vi "analyze-single-vi.vi"(0 "GObj引用句柄":refnum<vi>, 1 "type":string="subvi", 2 "context":string[][](array[string]), 3 "json_input":string caption="<JSON>Object") -> (7 "<JSON> 3":string caption="<JSON>")   [LabVIEW 2020]
panel:
  out "VI路径":path
  out "所有对象[] 2":string[][](table)
  out "数组 2":string[](array[string])
  in  "字符串":string="data\\"
  out "添加的路径":path
  out "x > 0?":bool
  out "布尔":bool
  in  "路径":path=path "C:/Users/Fred/Desktop/LabAI"
  in  "排除路径":string[](array[string])=["E:\\LabVIEW\\32-bit\\LabVIEW 2020"]
  in  "Path to Entrance VI":path=path "C:/Users/Fred/Desktop/LabAI/main.vi"
  # "C:\\Users\\Fred\\Desktop\\LabAI\\get_status_code.vi"
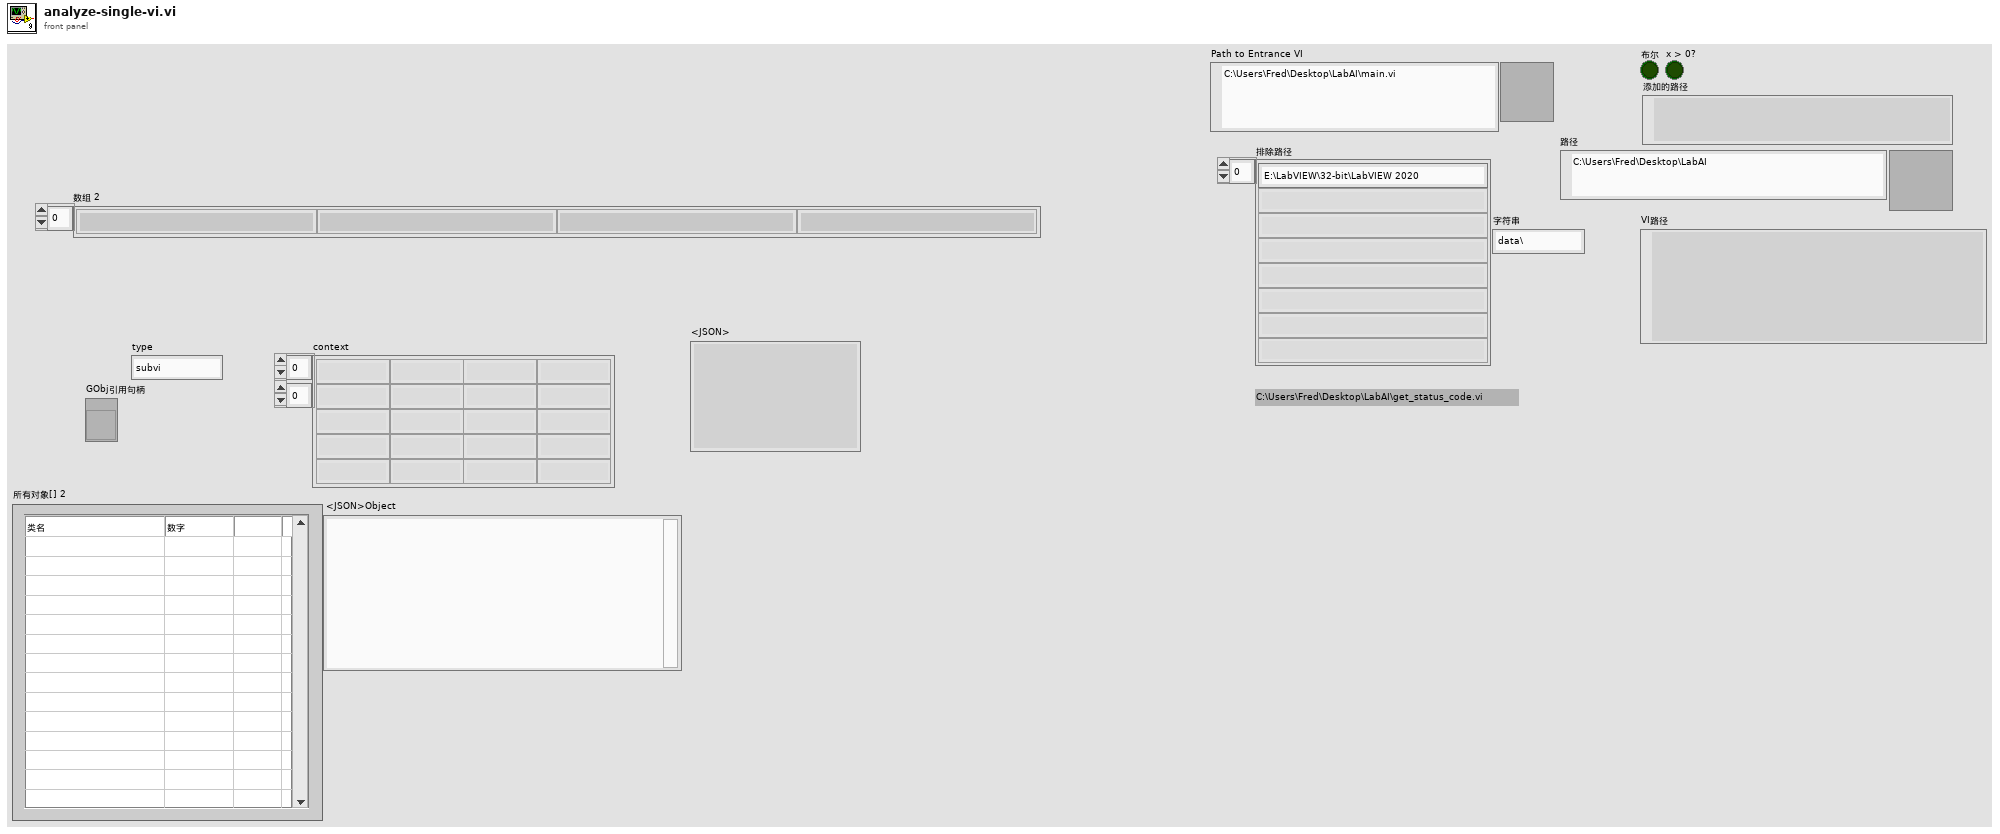
[diagram p1: front panel]
types:
  T1 = enum16{"open", "replace", "create", "open or create", "replace or create", "replace or create with confirmation"}
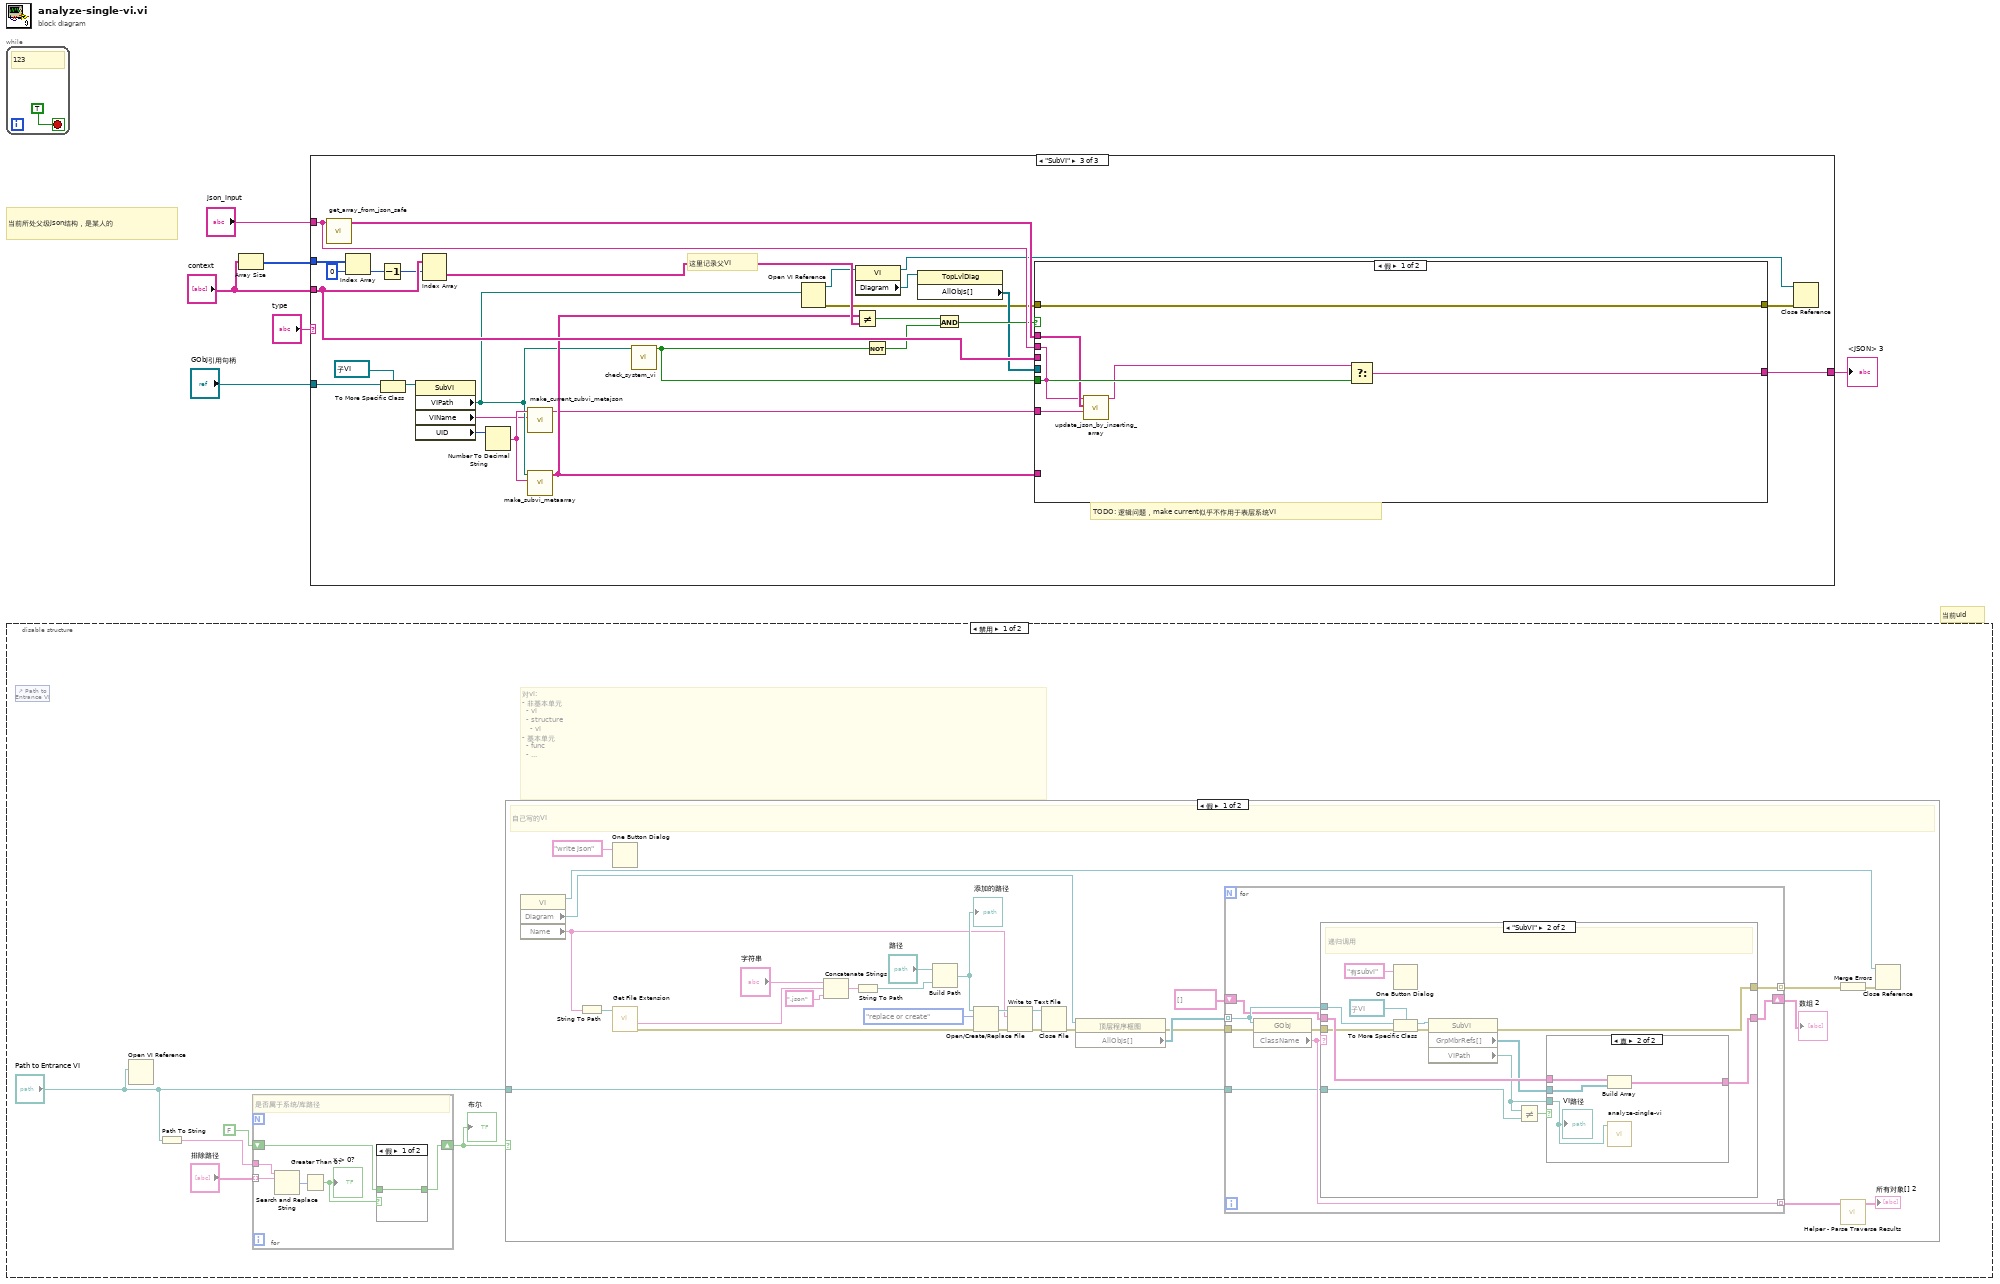
[diagram p0: block diagram]
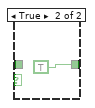
[diagram p2: hidden frame]
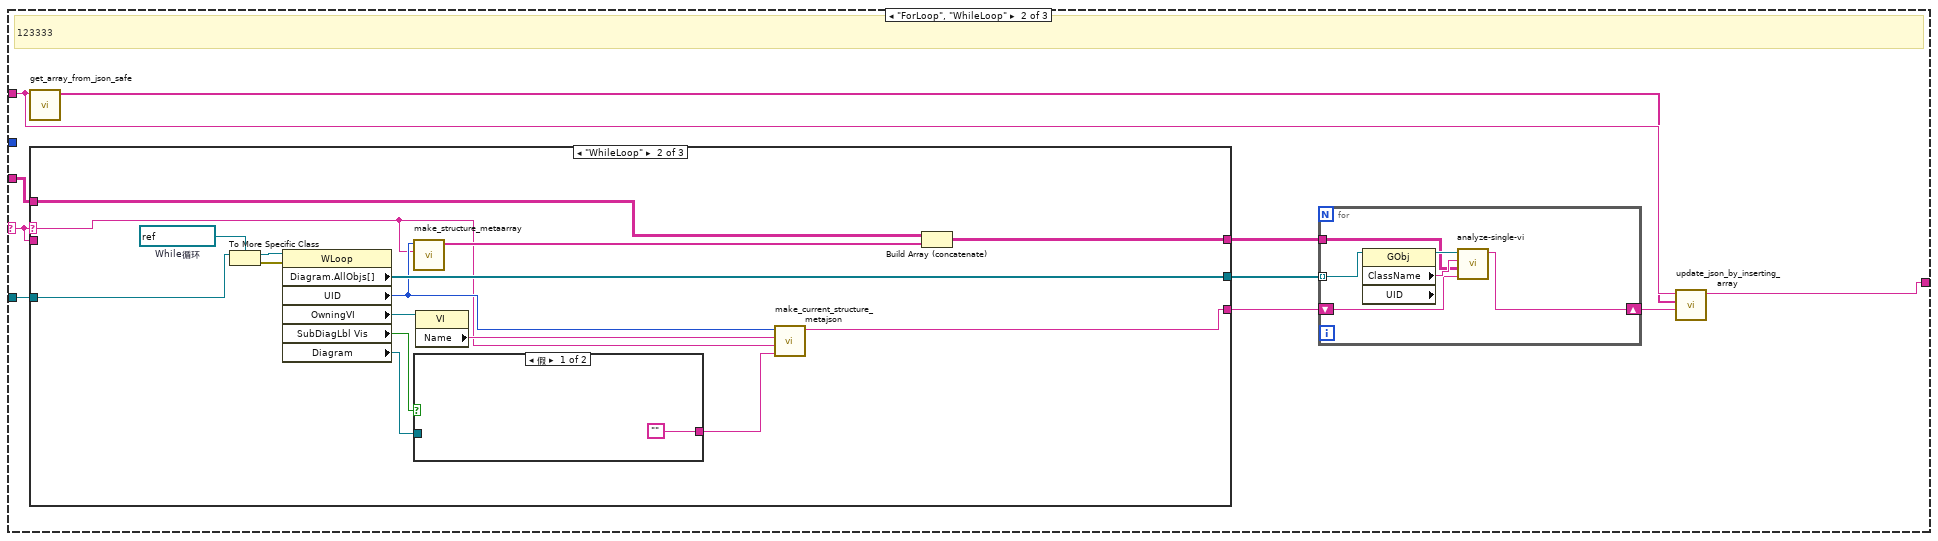
[diagram p8: hidden frame]
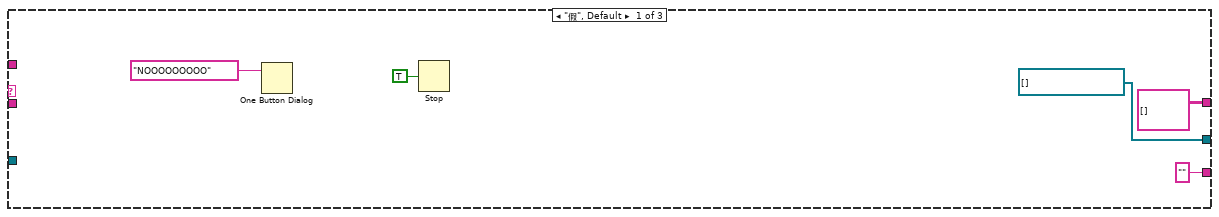
[diagram p9: hidden frame]
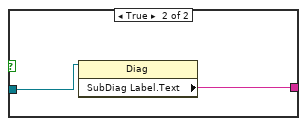
[diagram p10: hidden frame]
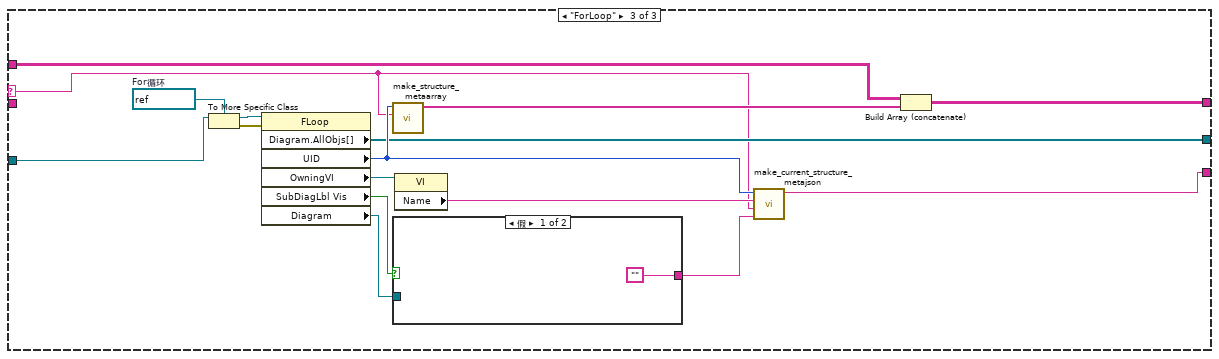
[diagram p11: hidden frame]
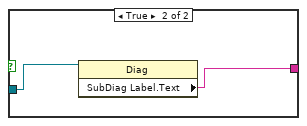
[diagram p12: hidden frame]
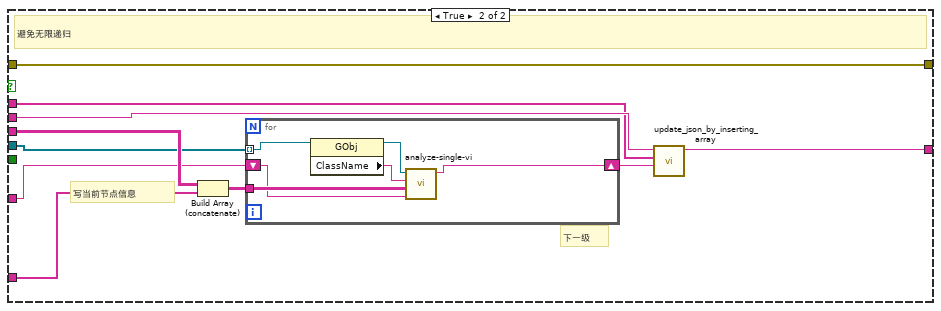
[diagram p13: hidden frame]
diagram:
  # "当前uid"
  # "当前所处父级json结构，是某人的"
  n1 = while {
    stop <- TRUE stop-if-true
    # "123"
  }
  n2 = disable-structure shown="禁用" {
    frame Disabled {
      # "对vi:\n- 非基本单元\n  - vi\n  - structure\n    - vi\n- 基本单元\n  - func\n  - ..."
      n3 = control-ref of="Path to Entrance VI"() -> ()  [unwired: 1 out]
      n4 = Open VI Reference(vi path="Path to Entrance VI") -> ()  [unwired: 5 in, 2 out]
      n5 = Path To String(path="Path to Entrance VI") -> (string=w11:string)
      n6 = for {
        tunnel: "排除路径" -> [w18] mode=indexing
        tunnel: w11 -> [w17]
        shift-right: [w13] -> w9
        shift-left: FALSE -> [w14]
        # "是否属于系统/库路径"
        n7 = Search and Replace String(input string=w17, search string=w18) -> (number of replacements=w16:i32)  [unwired: 6 in, 3 out]
        n8 = Greater Than 0?(x=w16) -> (x > 0?=w15:bool)
        "x > 0?" <- w15
        n9 = case shown="假" w15 {
          tunnel: [w19 TRUE] -> w13
          tunnel: w14 -> [w19 _]
          frame False {
          }
          frame True {
          }
        }
      }
      "布尔" <- w9
      n10 = case shown="假" w9 {
        tunnel: "Path to Entrance VI" -> [w21 _]
        frame False {
          # "自己写的VI"
          n11 = property class="VI"() -> (reference out=w31:refnum<vi>, "Diagram"=w33:refnum<vi>, "Name"=w29:string)  [unwired: 2 in, 1 out]
          n12 = String To Path(string=w29) -> (path=w30:path)
          n13 = One Button Dialog(message="write json" ("消息")) -> ()  [unwired: 1 in, 1 out]
          n14 = call <vilib>:"Get File Extension.vi"("file"=w30) -> ("error out"=w26:errorcluster, "filename without extension"=w41:string)  [unwired: 6 in, 3 out]
          n15 = Concatenate Strings("字符串", w41, ".json" ("字符串")) -> (w42:string)
          n16 = String To Path(string=w42) -> (path=w38:path)
          n17 = Build Path(base path="路径", name or relative path=w38) -> (appended path=w48:path)
          "添加的路径" <- w48
          n18 = Open/Create/Replace File(file path (use dialog)=w48, error in=w26, operation (0:open)=T1."replace or create" ("操作(0:open)")) -> (refnum out=w47:refnum<file>, error out=w25:errorcluster)  [unwired: 3 in, 1 out]
          n19 = Write to Text File(file (use dialog)=w47, text=w29, error in=w25) -> (refnum out=w46:refnum<file>, error out=w23:errorcluster)  [unwired: 1 in, 1 out]
          n20 = Close File(refnum=w46, error in=w23) -> (error out=w22:errorcluster)  [unwired: 1 out]
          n21 = property class="顶层程序框图"(reference=w33, error in=w22) -> (error out=w28:errorcluster, "AllObjs[]"=w32:refnum<vi>[])  [unwired: 1 out]
          n22 = for {
            tunnel: w32 -> [w55] mode=indexing
            tunnel: [w56] -> w34 mode=indexing
            shift-right: [w54] -> w37
            shift-left: string[] [] -> [w53]
            tunnel: w28 -> [w52]
            tunnel: [w50] -> w27 mode=indexing
            tunnel: w21 -> [w49]
            n23 = property class="GObj"(reference=w55, error in=w52) -> (error out=w51:errorcluster, "ClassName"=w56:string)  [unwired: 1 out]
            n24 = case shown="\"SubVI\"" w56 {
              tunnel: w55 -> [_ w69]
              tunnel: [w58 w68] -> w54
              tunnel: w53 -> [w58 w67]
              tunnel: w51 -> [w57 w66]
              tunnel: [w57 w64] -> w50
              tunnel: w49 -> [_ w60]
              frame "假", Default {
              }
              frame "SubVI" {
                # "递归调用"
                n25 = One Button Dialog(message="有subvi" ("消息")) -> ()  [unwired: 1 in, 1 out]
                n26 = To More Specific Class(target class=refnum<vi> refnum ("引用"), reference=w69, error in=w66) -> (specific class reference=w71:refnum<vi>, error out=w65:errorcluster)
                n27 = property class="SubVI"(reference=w71, error in=w65) -> (error out=w64:errorcluster, "GrpMbrRefs[]"=w63:refnum<vi>[], "VIPath"=w61:path)  [unwired: 1 out]
                n28 = Not Equal?(x=w61, y=w60) -> (x != y?=w62:bool)
                n29 = case shown="真" w62 {
                  tunnel: [w72 w76] -> w68
                  tunnel: w67 -> [w72 w75]
                  tunnel: w61 -> [_ w74]
                  tunnel: w63 -> [_ w73]
                  frame False {
                  }
                  frame True {
                    n30 = Build Array(w75, w73) -> (w76:string[][])
                    n31 = call "analyze-single-vi.vi"("Path to Entrance VI"=w74) -> ()  [unwired: 11 in]
                    "VI路径" <- w74
                  }
                }
              }
            }
          }
          "数组 2" <- w37
          n32 = Merge Errors(w27) -> (w24:errorcluster)
          n33 = call "Helper - Parse Traverse Results.vi"("遍历结果"=w34) -> ("解析结果"=→"所有对象[] 2":string[][])  [unwired: 10 in]
          n34 = Close Reference(reference=w31, error in (no error)=w24) -> ()  [unwired: 1 out]
        }
        frame True {
          # "系统路径不关心"
        }
      }
    }
    frame Enabled {
    }
  }
  n35 = Array Size(array="context") -> (size(s)=w2:i32[])
  n36 = case shown="\"SubVI\"" "type" {
    selector: "type" -> [_ w78 _]
    tunnel: "GObj引用句柄" -> [_ w87 w153]
    tunnel: "context" -> [_ w86 w164]
    tunnel: "json_input" -> [w77 w81 w159]
    tunnel: [w77 w82 w157] -> w3
    tunnel: w2 -> [_ _ w156]
    frame Default {
    }
    frame "ForLoop", "WhileLoop" {
      # "123333"
      n37 = call "get_array_from_json_safe.vi"("<JSON>输入"=w81) -> ("<JSON>输出"=w80:string[])  [unwired: 10 in]
      n38 = case shown="\"WhileLoop\"" w78 {
        selector: w78 -> [_ w96 w115]
        tunnel: w87 -> [_ w108 w121]
        tunnel: w86 -> [_ w107 w122]
        tunnel: [refnum<vi>[] [] ("Diagram.AllObjs[]") w103 w118] -> w85
        tunnel: [string[][] [] w101 w120] -> w84
        tunnel: ["" ("curr_while_metajson") w100 w119] -> w79
        tunnel: w78 -> [_ _ _]
        frame "假", Default {
          n39 = One Button Dialog(message="NOOOOOOOOO" ("消息")) -> ()  [unwired: 1 in, 1 out]
          n40 = Stop(stop? (T)=TRUE ("停止？(T)")) -> ()
        }
        frame "WhileLoop" {
          w104 = refnum<vi> refnum  # While循环
          n41 = To More Specific Class(target class=w104, reference=w108) -> (specific class reference=w106:refnum<vi>, error out=w105:errorcluster)  [unwired: 1 in]
          n42 = property class="WLoop"(reference=w106, error in=w105) -> ("Diagram.AllObjs[]"=w103:refnum<vi>[], "UID"=w99:i32, "OwningVI"=w98:refnum<vi>, "SubDiagLbl Vis"=w95:bool, "Diagram"=w94:refnum<vi>)  [unwired: 2 out]
          n43 = call "make_structure_metaarray.vi"("structure_type"=w96, "UID"=w99) -> ("数组"=w102:string[])  [unwired: 9 in]
          n44 = case shown="假" w95 {
            tunnel: ["" ("SubDiag Label.Text") w111] -> w93
            tunnel: w94 -> [_ w110]
            frame False {
            }
            frame True {
              n45 = property class="Diag"(reference=w110) -> ("SubDiag Label.Text"=w111:string)  [unwired: 1 in, 2 out]
            }
          }
          n46 = property class="VI"(reference=w98) -> ("Name"=w97:string)  [unwired: 1 in, 2 out]
          n47 = call "make_current_structure_metajson.vi"("structure_label"=w93, "type"=w96, "VIName"=w97, "UID"=w99) -> ("curr_while_metajson"=w100:string)  [unwired: 7 in]
          n48 = Build Array (concatenate)(w107, w102) -> (w101:string[][])
        }
        frame "ForLoop" {
          w125 = refnum<vi> refnum  # For循环
          n49 = To More Specific Class(target class=w125, reference=w121) -> (specific class reference=w127:refnum<vi>, error out=w126:errorcluster)  [unwired: 1 in]
          n50 = property class="FLoop"(reference=w127, error in=w126) -> ("Diagram.AllObjs[]"=w118:refnum<vi>[], "UID"=w123:i32, "OwningVI"=w117:refnum<vi>, "SubDiagLbl Vis"=w112:bool, "Diagram"=w114:refnum<vi>)  [unwired: 2 out]
          n51 = call "make_structure_metaarray.vi"("structure_type"=w115, "UID"=w123) -> ("数组"=w124:string[])  [unwired: 9 in]
          n52 = case shown="假" w112 {
            tunnel: w114 -> [_ w130]
            tunnel: ["" ("SubDiag Label.Text") w129] -> w113
            frame False {
            }
            frame True {
              n53 = property class="Diag"(reference=w130) -> ("SubDiag Label.Text"=w129:string)  [unwired: 1 in, 2 out]
            }
          }
          n54 = property class="VI"(reference=w117) -> ("Name"=w116:string)  [unwired: 1 in, 2 out]
          n55 = call "make_current_structure_metajson.vi"("structure_label"=w113, "type"=w115, "VIName"=w116, "UID"=w123) -> ("curr_while_metajson"=w119:string)  [unwired: 7 in]
          n56 = Build Array (concatenate)(w122, w124) -> (w120:string[][])
        }
      }
      n57 = for {
        tunnel: w84 -> [w133]
        tunnel: w85 -> [w134] mode=indexing
        shift-right: [w131] -> w83
        shift-left: w79 -> [w132]
        n58 = property class="GObj" props=["ClassName", "UID"](reference=w134) -> (reference out=w135:refnum<vi>, "ClassName"=w136:string)  [unwired: 1 in, 2 out]
        n59 = call "analyze-single-vi.vi"("GObj引用句柄"=w135, "type"=w136, "context"=w133, "json_input"=w132) -> ("<JSON> 3"=w131:string)  [unwired: 6 in]
      }
      n60 = call "update_json_by_inserting_array.vi"("json_to_insert_to_array(from recursive output)"=w83, "ori_json_array"=w80, "original_json"=w81) -> ("<JSON>输出"=w82:string)  [unwired: 8 in]
    }
    frame "SubVI" {
      # "TODO: 逻辑问题，make current似乎不作用于表层系统VI"
      # "这里记录父VI"
      n61 = call "get_array_from_json_safe.vi"("<JSON>输入"=w159) -> ("<JSON>输出"=w158:string[])  [unwired: 10 in]
      n62 = Index Array(array=w156, index=0 ("索引")) -> (element=w162:i32)
      n63 = Decrement(x=w162) -> (x-1=w151:i32)
      n64 = To More Specific Class(target class=refnum<vi> refnum ("引用"), reference=w153) -> (specific class reference=w152:refnum<vi>)  [unwired: 1 in, 1 out]
      n65 = property class="SubVI"(reference=w152) -> ("VIPath"=w146:path, "VIName"=w138:string, "UID"=w140:i32)  [unwired: 1 in, 2 out]
      n66 = Index Array(array=w164, index (row)=w151) -> (element=w161:string[])  [unwired: 1 in]
      n67 = Number To Decimal String(number=w140) -> (decimal integer string=w155:string)  [unwired: 1 in]
      n68 = call "make_current_subvi_metajson.vi"("VIName"=w138, "uid"=w155) -> ("<JSON>"=w137:string)  [unwired: 9 in]
      n69 = call "make_subvi_metaarray.vi"("UID"=w155, "VIPath"=w146) -> ("数组"=w160:string[])  [unwired: 9 in]
      n70 = call "check_system_vi.vi"("VIPath"=w146) -> ("布尔 2"=w139:bool)  [unwired: 9 in, 1 out]
      n71 = Open VI Reference(vi path=w146) -> (vi reference=w147:refnum<vi>, error out=w143:errorcluster)  [unwired: 5 in]
      n72 = property class="VI"(reference=w147) -> (reference out=w141:refnum<vi>, "Diagram"=w145:refnum<vi>)  [unwired: 1 in, 1 out]
      n73 = Not Equal?(x=w160, y=w161) -> (x != y?=w149:bool)
      n74 = Not(x=w139) -> (.not. x?=w148:bool)
      n75 = property class="TopLvlDiag"(reference=w145) -> ("AllObjs[]"=w144:refnum<vi>[])  [unwired: 1 in, 2 out]
      n76 = And(x=w149, y=w148) -> (x .and. y?=w150:bool)
      n77 = case shown="假" w150 {
        tunnel: w164 -> [_ w180]
        tunnel: w160 -> [_ w179]
        tunnel: w159 -> [w166 w178]
        tunnel: w158 -> [w168 w177]
        tunnel: [w165 w175] -> w157
        tunnel: w144 -> [_ w174]
        tunnel: [w171 w173] -> w142
        tunnel: w143 -> [w171 w173]
        tunnel: w139 -> [w170 _]
        tunnel: w137 -> [w169 w172]
        frame False {
          n78 = call "update_json_by_inserting_array.vi"("json_to_insert_to_array(from recursive output)"=w169, "ori_json_array"=w168, "original_json"=w166) -> ("<JSON>输出"=w167:string)  [unwired: 8 in]
          n79 = Select(t=w167, s=w170, f=w166) -> (s? t:f=w165:string)
        }
        frame True {
          # "写当前节点信息"
          # "下一级"
          # "避免无限递归"
          n80 = Build Array (concatenate)(w180, w179) -> (w181:string[][])
          n81 = for {
            tunnel: w181 -> [w185]
            shift-right: [w183] -> w176
            shift-left: w172 -> [w184]
            tunnel: w174 -> [w182] mode=indexing
            n82 = property class="GObj"(reference=w182) -> (reference out=w186:refnum<vi>, "ClassName"=w187:string)  [unwired: 1 in, 1 out]
            n83 = call "analyze-single-vi.vi"("GObj引用句柄"=w186, "type"=w187, "context"=w185, "json_input"=w184) -> ("<JSON> 3"=w183:string)  [unwired: 6 in]
          }
          n84 = call "update_json_by_inserting_array.vi"("json_to_insert_to_array(from recursive output)"=w176, "ori_json_array"=w177, "original_json"=w178) -> ("<JSON>输出"=w175:string)  [unwired: 8 in]
        }
      }
      n85 = Close Reference(reference=w141, error in (no error)=w142) -> ()  [unwired: 1 out]
    }
  }
  "<JSON> 3" <- w3
